vi "Disconnect.vi"(8 "error in (no error)":errorcluster, 11 "34401 in":refnum<class "34401.lvclass">) -> (0 "error out":errorcluster, 3 "34401 out":refnum<class "34401.lvclass">)   [LabVIEW 2018, in "34401.lvlib" / "34401.lvclass"]
uses:
  34401.lvclass
  34401.lvclass/34401.ctl
  <instrlib>/Agilent 34401/Agilent 34401.lvlib
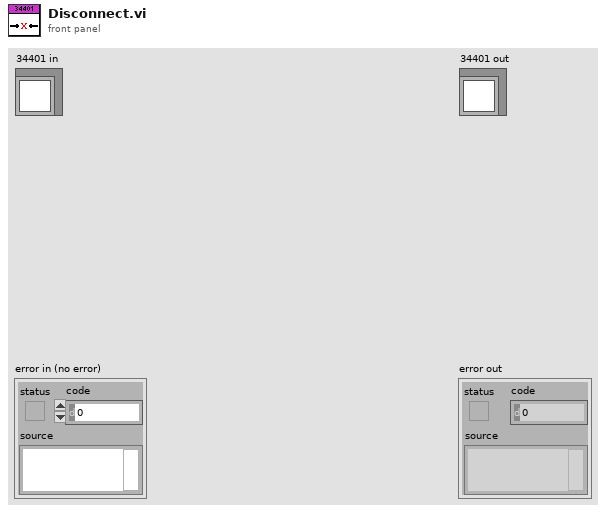
[diagram p1: front panel]
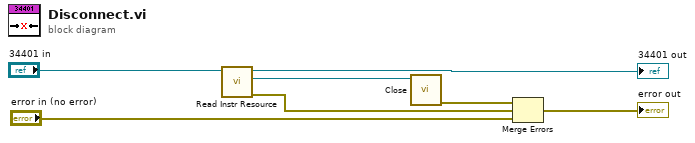
[diagram p0: block diagram]
diagram:
  n1 = call "Read Instr Resource.vi"("34401 in"="34401 in") -> ("error out"=w4:errorcluster, "Instr Resource"=w6:refnum<visa-resource-name>, "34401 out"=→"34401 out":refnum<class "34401.lvclass">)  [unwired: 8 in]
  n2 = call <instrlib>:"Close.vi"("VISA resource name"=w6) -> ("error out"=w5:errorcluster)  [unwired: 10 in]
  n3 = Merge Errors(w5, w4, "error in (no error)") -> (→"error out":errorcluster)
